vi "LCR Meter LIST Measurement.vi"() -> ()   [LabVIEW 2021, in "LCR Meter.lvlib"]
doc: "This example shows simple LIST measurement."
uses:
  LCR Meter.lvlib
panel:
  in  "Wait to read value and stop(5000)":u32=5000
  out "Spot 10":string
  out "Spot 9":string
  out "Spot 8":string
  out "Spot 7":string
  out "Spot 6":string
  out "Spot 5":string
  out "Spot 4":string
  out "Spot 3":string
  out "Spot 2":string
  out "Spot 1":string
  in  "Serial Settings:Baud Rate":u32(ring)=115200 items=["9600"=9600, "38400"=38400, "57600"=57600, "115200"=115200]
  in  "VISA resource name":refnum<visa-resource-name>
  # "ms"
  # "Note : Freq in 1KHz"
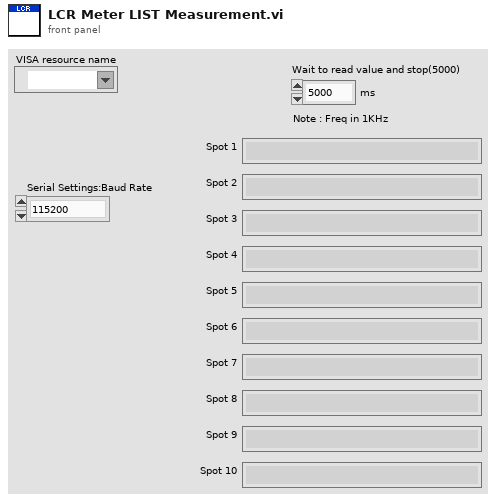
[diagram p1: front panel]
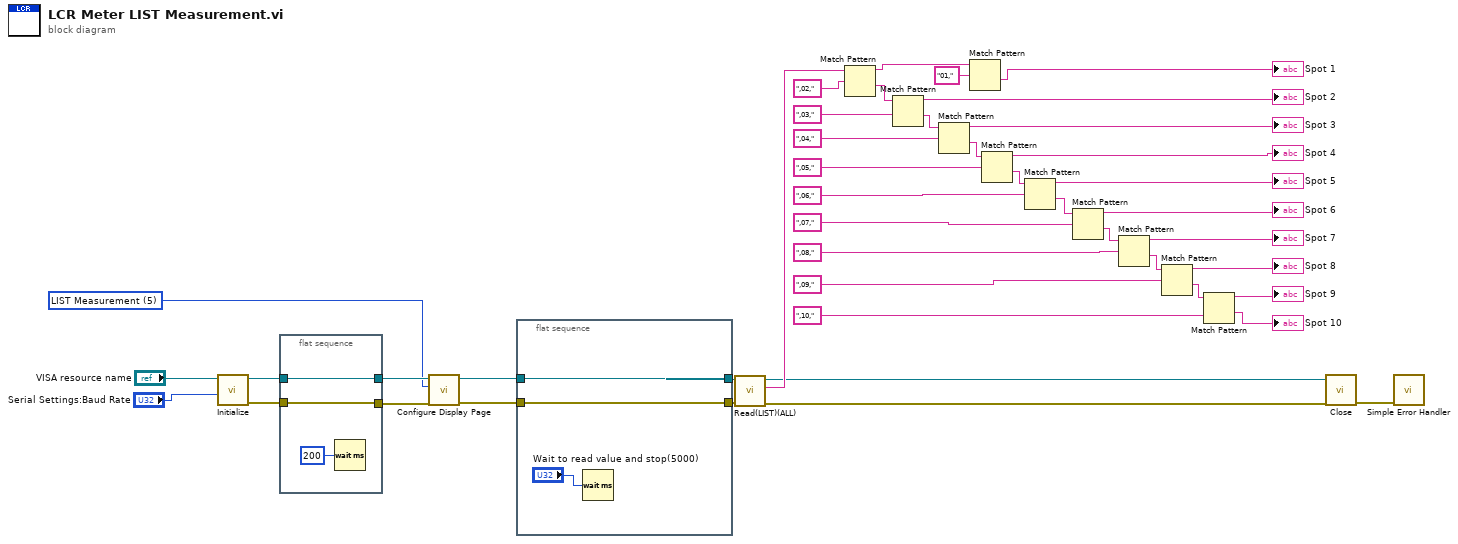
[diagram p0: block diagram]
diagram:
  w37 = u16 5 items=["Measurement", "Measurement Setup", "BIN Measurement", "BIN Count", "BIN Setup", "LIST Measurement", "LIST Setup", "CORRECTION", "CATALOG", "ENLARGE", "System Config", "System Information"] ("Display Page")
  n1 = call "Initialize.vi"("Serial Settings:Baud Rate"="Serial Settings:Baud Rate", "VISA resource name"="VISA resource name") -> ("error out"=w39:errorcluster, "VISA resource name out"=w41:refnum<visa-resource-name>)  [unwired: 7 in, 1 out]
  n2 = flat-sequence {
    tunnel: w41 -> [w47]
    tunnel: [w47] -> w40
    tunnel: [w46] -> w38
    tunnel: w39 -> [w46]
    frame #0 {
      n3 = Wait (ms)(milliseconds to wait=u32 200) -> ()  [unwired: 1 out]
    }
  }
  n4 = call "Configure Display Page.vi"("error in"=w38, "Display Page"=w37, "VISA resource name"=w40) -> ("error out"=w5:errorcluster, "VISA resource name out"=w6:refnum<visa-resource-name>)  [unwired: 7 in]
  n5 = flat-sequence {
    tunnel: w6 -> [w50]
    tunnel: w5 -> [w49]
    tunnel: [w50] -> w4
    tunnel: [w49] -> w3
    frame #0 {
      n6 = Wait (ms)(milliseconds to wait="Wait to read value and stop(5000)") -> ()  [unwired: 1 out]
    }
  }
  n7 = call "Read(LIST)(ALL).vi"("error in"=w3, "VISA resource name"=w4) -> ("error out"=w1:errorcluster, "Result"=w7:string, "VISA resource name out"=w2:refnum<visa-resource-name>)  [unwired: 7 in]
  n8 = Match Pattern(string=w7, regular expression=",02,") -> (before substring=w34:string, after substring=w9:string)  [unwired: 1 in, 2 out]
  n9 = Match Pattern(string=w9, regular expression=",03,") -> (before substring=→"Spot 2":string, after substring=w10:string)  [unwired: 1 in, 2 out]
  n10 = Match Pattern(string=w10, regular expression=",04,") -> (before substring=→"Spot 3":string, after substring=w12:string)  [unwired: 1 in, 2 out]
  n11 = Match Pattern(string=w34, regular expression="01,") -> (after substring=→"Spot 1":string)  [unwired: 1 in, 3 out]
  n12 = Match Pattern(string=w12, regular expression=",05,") -> (before substring=→"Spot 4":string, after substring=w18:string)  [unwired: 1 in, 2 out]
  n13 = Match Pattern(string=w18, regular expression=",06,") -> (before substring=→"Spot 5":string, after substring=w15:string)  [unwired: 1 in, 2 out]
  n14 = Match Pattern(string=w15, regular expression=",07,") -> (before substring=→"Spot 6":string, after substring=w16:string)  [unwired: 1 in, 2 out]
  n15 = Match Pattern(string=w16, regular expression=",08,") -> (before substring=→"Spot 7":string, after substring=w17:string)  [unwired: 1 in, 2 out]
  n16 = Match Pattern(string=w17, regular expression=",09,") -> (before substring=→"Spot 8":string, after substring=w23:string)  [unwired: 1 in, 2 out]
  n17 = Match Pattern(string=w23, regular expression=",10,") -> (before substring=→"Spot 9":string, after substring=→"Spot 10":string)  [unwired: 1 in, 2 out]
  n18 = call "Close.vi"("error in (no error)"=w1, "VISA resource name"=w2) -> ("error out"=w42:errorcluster)  [unwired: 9 in]
  n19 = call <vilib>:"Simple Error Handler.vi"("error in (no error)"=w42) -> ()  [unwired: 4 in, 5 out]
